vi "NI 機器視覺_存檔.vi"() -> ()   [LabVIEW 2019]
panel:
  in  "stop":bool
  out "Image":T1(plugin-control)
  in  "OK Button":bool
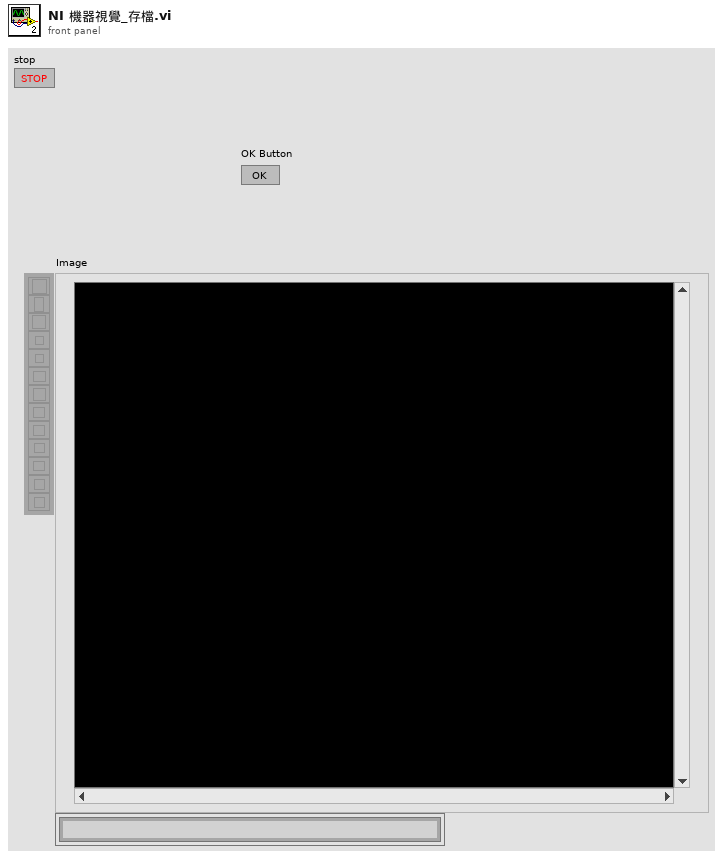
[diagram p1: front panel]
types:
  T1 = typedef "IMAQ Image.ctl" = refnum<image>
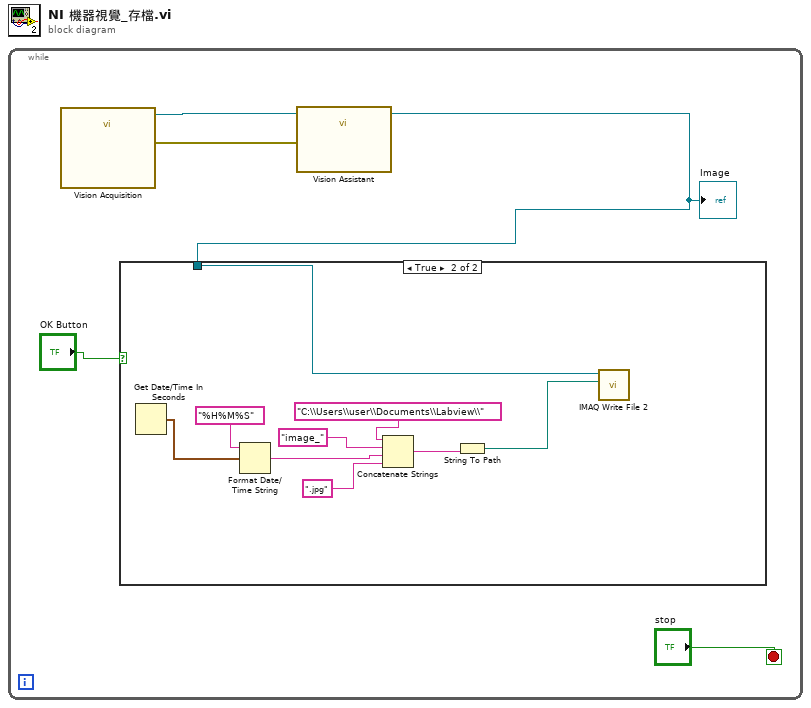
[diagram p0: block diagram]
diagram:
  n1 = while {
    stop <- "stop" stop-if-true
    n2 = call "Vision Acquisition"() -> ("Image Out"=w5:T1, "error out"=w4:errorcluster)  [unwired: 25 in, 1 out]
    n3 = call "Vision Assistant"("Image In"=w5, "error in"=w4) -> ("Image Out"=w2:T1)  [unwired: 24 in, 1 out]
    "Image" <- w2
    n4 = case shown="True" "OK Button" {
      tunnel: w2 -> [_ w14]
      frame False {
      }
      frame True {
        n5 = Get Date/Time In Seconds() -> (seconds since 1Jan1904=w13:timestamp)
        n6 = Format Date/Time String(time format string (%c)="%H%M%S", seconds (now)=w13) -> (date/time string=w10:string)  [unwired: 1 in]
        n7 = Concatenate Strings("C:\\Users\\user\\Documents\\Labview\\" ("string"), "image_" ("string"), w10, ".jpg" ("string")) -> (w7:string)
        n8 = String To Path(string=w7) -> (path=w6:path)
        n9 = call-poly "IMAQ Write File 2"("File Path"=w6, "Image"=w14) -> ()  [unwired: 8 in, 2 out]
      }
    }
  }
